vi "BitField_Read.vi"(5 "stop (In)":u8, 7 "start (In)":u8, 11 "value (In)":u32=7 format="%032b") -> (3 "sliced value (Out)":u32 format="%032b")   [LabVIEW 2014]
panel:
  out "value shifted right":u32 format="%032b"
  out "mask stop-start":u32 format="%032b"
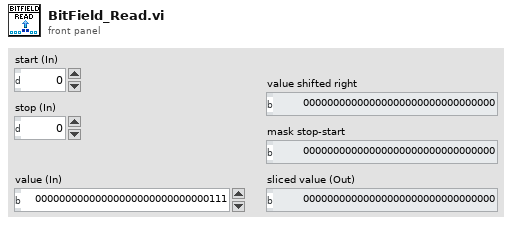
[diagram p1: front panel]
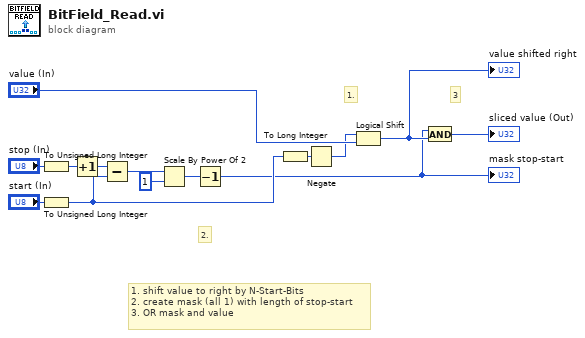
[diagram p0: block diagram]
diagram:
  # "1. shift value to right by N-Start-Bits\n2. create mask (all 1) with length of stop-start\n3. OR mask and value"
  # "3"
  # "2."
  # "1."
  n1 = To Unsigned Long Integer(number="stop (In)") -> (unsigned 32bit integer=w10:u32)
  n2 = To Unsigned Long Integer(number="start (In)") -> (unsigned 32bit integer=w7:u32)
  n3 = Increment(x=w10) -> (x+1=w1:u32)
  n4 = Subtract(x=w1, y=w7) -> (x-y=w8:u32)
  n5 = Scale By Power Of 2(n=w8, x=u32 1) -> (x*2^n=w9:u32)
  n6 = Decrement(x=w9) -> (x-1=w2:u32)
  "mask stop-start" <- w2
  n7 = To Long Integer(number=w7) -> (32bit integer=w3:i32)
  n8 = Negate(x=w3) -> (-x=w4:i32)
  n9 = Logical Shift(y=w4, x="value (In)") -> (x << y=w12:u32)
  "value shifted right" <- w12
  n10 = And(x=w2, y=w12) -> (x .and. y?=→"sliced value (Out)":u32)
